vi "Read configuration.vi"(8 "error in":errorcluster, 11 "Profibus Module editor node in":refnum<class "Profibus Module editor node.lvclass">) -> (0 "error out":errorcluster, 2 "TBM configuration out":refnum<class "NISE_CEF_serializable configuration.lvclass">, 3 "Profibus Module editor node out":refnum<class "Profibus Module editor node.lvclass">)   [LabVIEW 2013, in "Profibus Module editor node.lvclass"]
uses:
  Profibus Module editor node.lvclass
  <vilib>/NI/Configuration Framework/serializable configuration/NISE_CEF_serializable configuration.lvclass
  Profibus Module editor node.lvclass/Profibus Module editor node.ctl
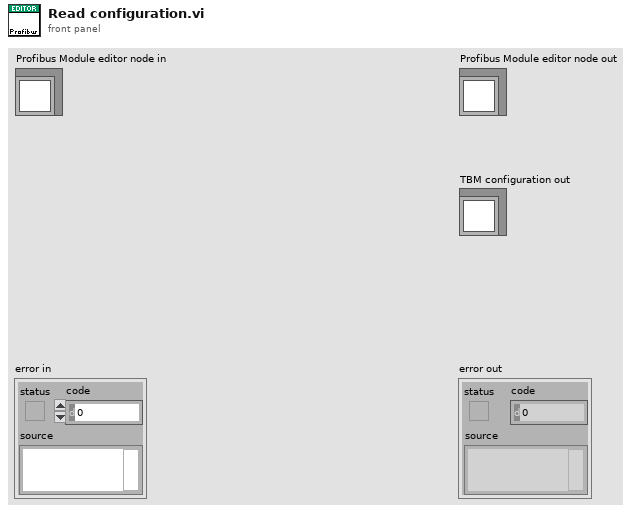
[diagram p1: front panel]
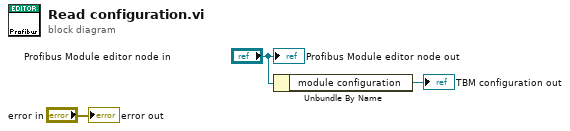
[diagram p0: block diagram]
diagram:
  n1 = Unbundle By Name("Profibus Module editor node in") -> ("module configuration"=→"TBM configuration out":refnum<class "Profibus Module configuration.lvclass">)
  "error out" <- "error in"
  "Profibus Module editor node out" <- "Profibus Module editor node in"
